vi "Stop Iterations.vi"(8 "error in (no error)":errorcluster, 11 "Iterator Actor in":refnum<class "Abstract Iterator Actor.lvclass">) -> (0 "error out":errorcluster, 3 "Iterator Actor out":refnum<class "Abstract Iterator Actor.lvclass">)   [LabVIEW 2021, in "Iterator Actor.lvlib" / "Abstract Iterator Actor.lvclass"]
doc: "Stops all the subsequent iterations."
uses:
  Abstract Iterator Actor.lvclass
  Abstract Iterator Actor.lvclass/Abstract Iterator Actor.ctl
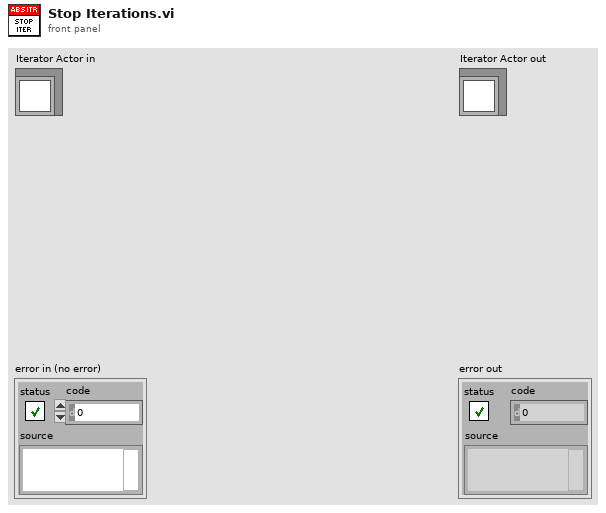
[diagram p1: front panel]
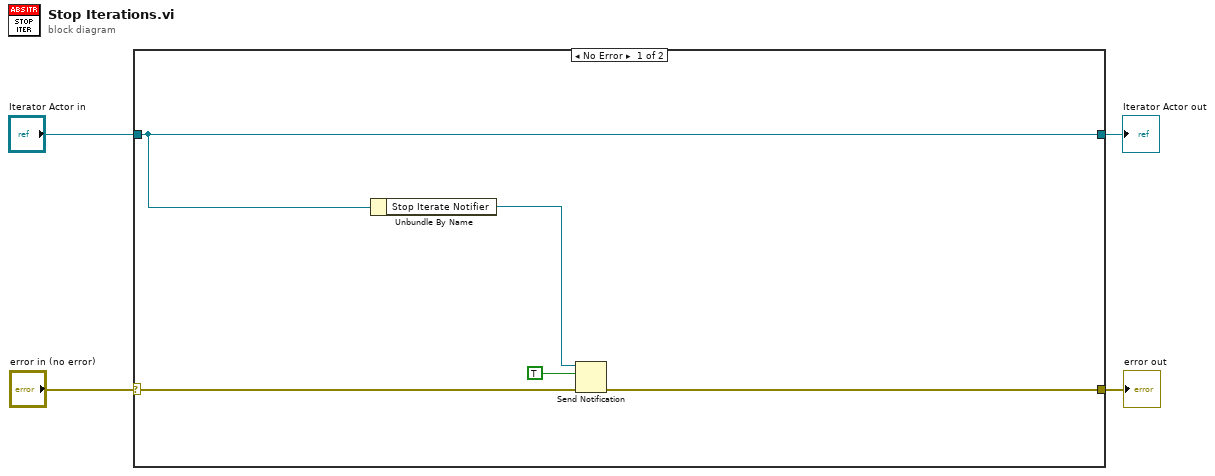
[diagram p0: block diagram]
diagram:
  n1 = case shown="No Error" "error in (no error)" {
    selector: "error in (no error)" -> [w8 w11]
    tunnel: [w9 w11] -> w3
    tunnel: [w5 w10] -> w1
    tunnel: "Iterator Actor in" -> [w5 w10]
    frame No Error {
      n2 = Unbundle By Name(w5) -> ("Stop Iterate Notifier"=w7:refnum<notifier>)
      n3 = Send Notification(notification=TRUE, notifier=w7, error in (no error)=w8) -> (error out=w9:errorcluster)  [unwired: 1 out]
    }
    frame Error {
    }
  }
  "error out" <- w3
  "Iterator Actor out" <- w1
